vi "ProbeMessageDefault.vi"(11 "Message":refnum<class "Message.lvclass">) -> (2 "Value String":string, 3 "Boolean":bool)   [LabVIEW 2017, in "LapDog.Messaging.v3.lvlib" / "Message.lvclass"]
uses:
  Message.lvclass
  Message.lvclass/Message.ctl
panel:
  out "Message Type":string
  out "Data":string
  out "Message Name":string
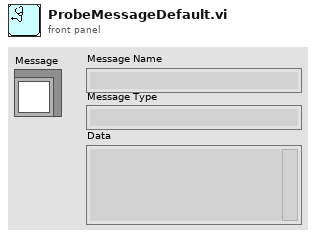
[diagram p1: front panel]
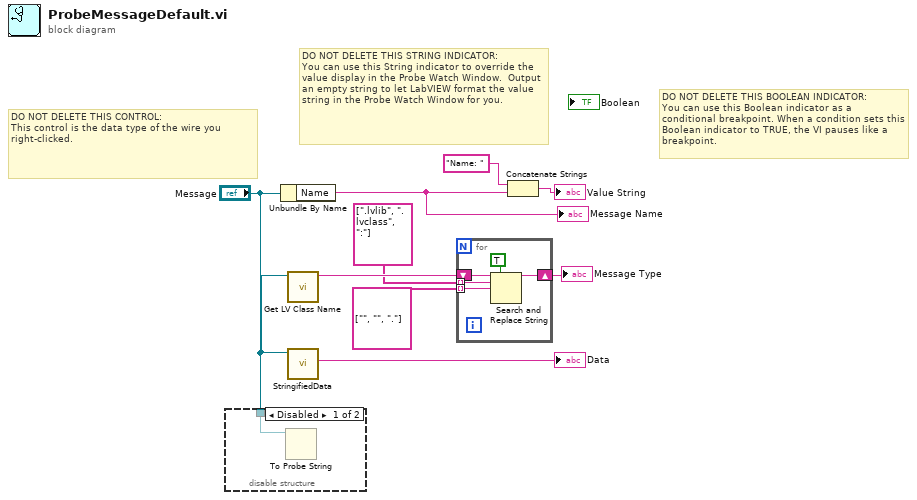
[diagram p0: block diagram]
diagram:
  # "DO NOT DELETE THIS STRING INDICATOR: \nYou can use this String indicator to override the value display in the Probe Watch Window.  Output an empty string to let LabVIEW format the value string in the Probe Watch Window for you."
  # "DO NOT DELETE THIS BOOLEAN INDICATOR: \nYou can use this Boolean indicator as a conditional breakpoint. When a condition sets this Boolean indicator to TRUE, the VI pauses like a breakpoint."
  # "DO NOT DELETE THIS CONTROL: \nThis control is the data type of the wire you right-clicked."
  n1 = disable-structure shown="Disabled" {
    disable-tunnel: "Message" -> [w10 _]
    frame Disabled {
      n2 = To Probe String(7:w10) -> ()  [unwired: 2 in, 2 out]
    }
    frame Enabled {
    }
  }
  n3 = Unbundle By Name("Message") -> ("Name"=w8:string)
  "Message Name" <- w8
  n4 = call <vilib>:"Get LV Class Name.vi"("object"="Message") -> ("class name"=w4:string)  [unwired: 9 in, 1 out]
  n5 = call-dynamic "StringifiedData.vi"("Message in"="Message") -> ("Stringified Data"=→"Data":string)  [unwired: 8 in, 2 out]
  n6 = for {
    shift-right: [w13] -> w1
    shift-left: w4 -> [w15]
    tunnel: string[] [".lvlib", ".lvclass", ":"] -> [w12] mode=indexing
    tunnel: string[] ["", "", "."] -> [w11] mode=indexing
    n7 = Search and Replace String(replace all?=TRUE ("replace all? (F)"), input string=w15, search string=w12, replace string=w11) -> (result string=w13:string)  [unwired: 4 in, 3 out]
  }
  "Message Type" <- w1
  n8 = Concatenate Strings("Name: " ("string"), w8) -> (→"Value String":string)
